vi "Init Attributes.vi"(10 "Attributes":T1) -> (3 "Base Attributes out":refnum<class "Base Attributes.lvclass">)   [LabVIEW 2025, in "jettl.lvlib" / "Attributes.lvlib" / "Base Attributes.lvclass"]
uses:
  Base Attributes.lvclass
  Attributes.ctl
  Attributes/Attributes.lvclass
  Refs/Refs.lvclass
  Transport/Transport/Transport.lvclass
  Spawn.ctl
  Msg Set.ctl
  Msg/Msg.lvclass
  Actor/Actor.lvclass
  Actor.ctl
  Base Attributes.lvclass/Base Attributes.ctl
  jettl.lvlib
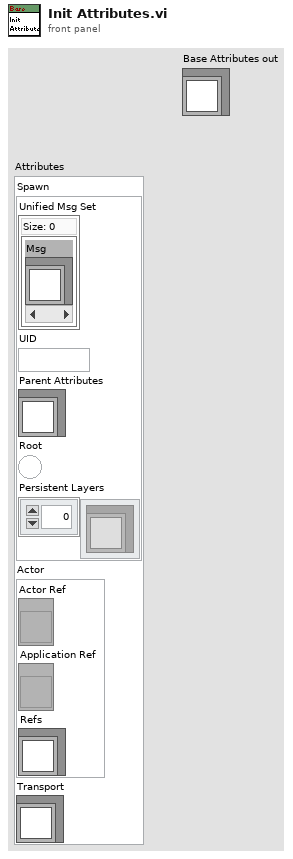
[diagram p1: front panel]
types:
  T1 = typedef "jettl.lvlib/Attributes.ctl" = cluster{"Spawn":T2, "Actor":T4, "Transport":refnum<class "Transport.lvclass">}
  T2 = typedef "jettl.lvlib/Spawn.ctl" = cluster{"Unified Msg Set":T3, "UID":string, "Parent Attributes":refnum<class "Attributes.lvclass">, "Root":bool, "Persistent Layers":refnum<class "Actor.lvclass">[]}
  T3 = typedef "jettl.lvlib/Msg Set.ctl" = set{refnum<class "Msg.lvclass">}
  T4 = typedef "jettl.lvlib/Actor.ctl" = cluster{"Actor Ref":refnum<vi>, "Application Ref":refnum<vi>, "Refs":refnum<class "Refs.lvclass">}
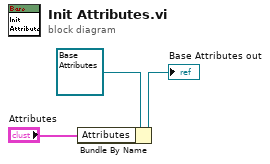
[diagram p0: block diagram]
diagram:
  n1 = Bundle By Name(cluster=refnum<class "Base Attributes.lvclass"> refnum ("Base Attributes in"), "Attributes"="Attributes") -> (→"Base Attributes out":refnum<class "Base Attributes.lvclass">)
